vi "FlatToRichgoogle_protobuf_Empty.vi"(5 "OutputClusterType":T1, 11 "InputCluster":T2) -> (3 "OutputCluster":T1)   [LabVIEW 2023, in "Generated_server.lvlib"]
uses:
  Generated_server.lvlib
  google_protobuf_Empty_Flat.ctl
  google_protobuf_Empty.ctl
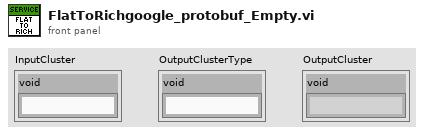
[diagram p1: front panel]
types:
  T1 = typedef "Generated_server.lvlib/google_protobuf_Empty.ctl" = cluster{"void":string}
  T2 = typedef "Generated_server.lvlib/google_protobuf_Empty_Flat.ctl" = cluster{"void":string}
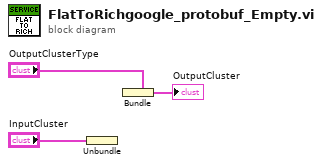
[diagram p0: block diagram]
diagram:
  n1 = Unbundle "Unbundle"("InputCluster") -> ()  [unwired: 1 out]
  n2 = Bundle "Bundle"(cluster="OutputClusterType") -> (→"OutputCluster":T1)  [unwired: 1 in]
